vi "mtg reader - get timestamp from filename.vi"(11 "name":string="20250806 - 0944.txt") -> (0 "offset":i32, 1 "hourly file":bool, 3 "Time Stamp":timestamp=timestamp(3837311040 s since 1904-01-01))   [LabVIEW 2025]
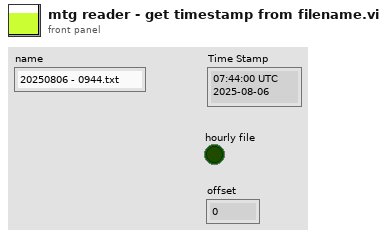
[diagram p1: front panel]
types:
  T1 = cluster{"second":i32, "minute":i32, "hour":i32, "day of month":i32, "month":i32, "year":i32, "day of week":i32, "day of year":i32, "is DST":i32}
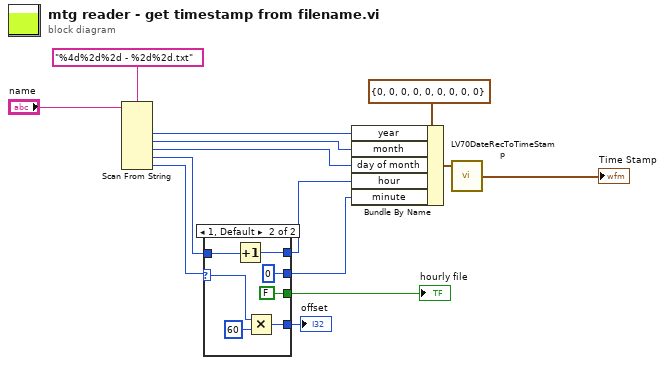
[diagram p0: block diagram]
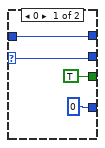
[diagram p2: hidden frame]
diagram:
  n1 = Scan From String(format string="%4d%2d%2d - %2d%2d.txt", input string="name") -> (output 1=w9:i32, output 2=w10:i32, output 3=w11:i32, output 4=w5:i32, output 5=w6:i32)  [unwired: 7 in, 3 out]
  n2 = case shown="1, Default" w6 {
    selector: w6 -> [w16 w20]
    tunnel: w5 -> [w18 w25]
    tunnel: [w18 w24] -> w4
    tunnel: [w16 0] -> w3
    tunnel: [TRUE FALSE] -> w2
    tunnel: [0 w19] -> w1
    frame 0 {
    }
    frame 1, Default {
      n3 = Increment(x=w25) -> (x+1=w24:i32)
      n4 = Multiply(x=w20, y=60) -> (x*y=w19:i32)
    }
  }
  "hourly file" <- w2
  "offset" <- w1
  n5 = Bundle By Name(cluster=T1 {"second"=0, "minute"=0, "hour"=0, "day of month"=0, "month"=0, "year"=0, "day of week"=0, "day of year"=0, "is DST"=0} ("date time rec"), "year"=w9, "month"=w10, "day of month"=w11, "hour"=w4, "minute"=w3) -> (w12:T1)
  n6 = call <vilib>:"LV70DateRecToTimeStamp.vi"("date time rec"=w12) -> ("Time Stamp"=→"Time Stamp":timestamp)
